vi "LV SciSDK TOF SPECTRUM START.vi"(0 "TOF Spectrum Name":string, 5 "Bin Width":u32, 7 "Start Delay":u32, 9 "Handle In":T2, 11 "error in (no error)":errorcluster) -> (10 "TOF Spectrum Handle Out":T1, 15 "error out":errorcluster)   [LabVIEW 2021]
uses:
  SciSDK_Labview.lvlib
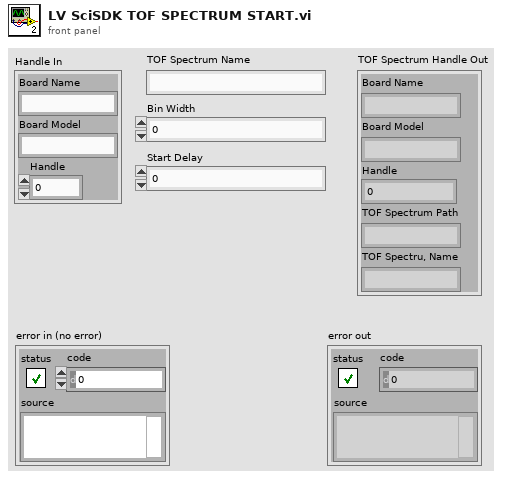
[diagram p1: front panel]
types:
  T1 = cluster{"Board Name":string, "Board Model":string, "Handle":u64, "TOF Spectrum Path":string, "TOF Spectru, Name":string}
  T2 = cluster{"Board Name":string, "Board Model":string, "Handle":u64}
  T3 = cluster{"Board Name":string, "Board Model":string, "Handle":u64, string, "TOF Spectrum Name":string}
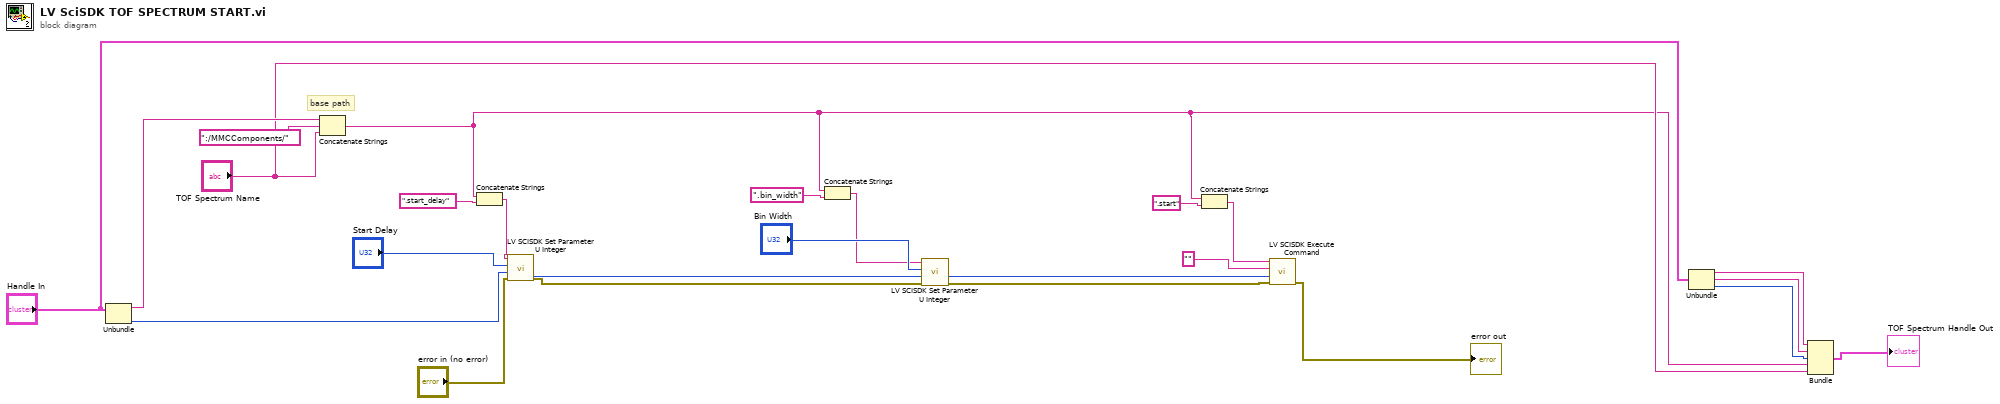
[diagram p0: block diagram]
diagram:
  # "base path"
  n1 = Unbundle("Handle In") -> ("Board Name"=w24:string, "Handle"=w10:u64)  [unwired: 1 out]
  n2 = Concatenate Strings(w24, ":/MMCComponents/" ("string"), "TOF Spectrum Name") -> (w1:string)
  n3 = Concatenate Strings(w1, ".start_delay" ("string")) -> (w13:string)
  n4 = call "LV SCISDK Set Parameter U Integer.vi"("error in (no error)"="error in (no error)", "handle"=w10, "value"="Start Delay", "Path"=w13) -> ("error out"=w8:errorcluster, "handle out"=w11:u64)  [unwired: 5 in, 1 out]
  n5 = Concatenate Strings(w1, ".bin_width" ("string")) -> (w12:string)
  n6 = call "LV SCISDK Set Parameter U Integer.vi"("error in (no error)"=w8, "handle"=w11, "value"="Bin Width", "Path"=w12) -> ("error out"=w7:errorcluster, "handle out"=w6:u64)  [unwired: 5 in, 1 out]
  n7 = Concatenate Strings(w1, ".start" ("string")) -> (w3:string)
  n8 = call "LV SCISDK Execute Command.vi"("error in (no error)"=w7, "handle"=w6, "value"="" ("concatenated string"), "Path"=w3) -> ("error out"=→"error out":errorcluster)  [unwired: 5 in, 2 out]
  n9 = Unbundle("Handle In") -> ("Board Name"=w20:string, "Board Model"=w19:string, "Handle"=w18:u64)
  n10 = Bundle("Board Name"=w20, "Board Model"=w19, "Handle"=w18, w1, "TOF Spectrum Name"="TOF Spectrum Name") -> (→"TOF Spectrum Handle Out":T3)  [unwired: 1 in]
